vi "Write Data Container.vi"(8 "error in (no error)":errorcluster, 10 "Data Container":T1 {"WaveformData"."StopTime" format="%<%x %.3X>T"; "WaveformData"."StartTime" format="%<%x %.3X>T"}, 11 "Task_Abstr in":refnum<class "Task_Abstr.lvclass">) -> (0 "error out":errorcluster, 3 "Task_Abstr out":refnum<class "Task_Abstr.lvclass">)   [LabVIEW 2025, in "Task_Abstr.lvlib" / "Task_Abstr.lvclass"]
uses:
  Task_Abstr.lvclass
  DataContainer.ctl
  WaveformData.ctl
  Task_Abstr.lvclass/Task_Abstr.ctl
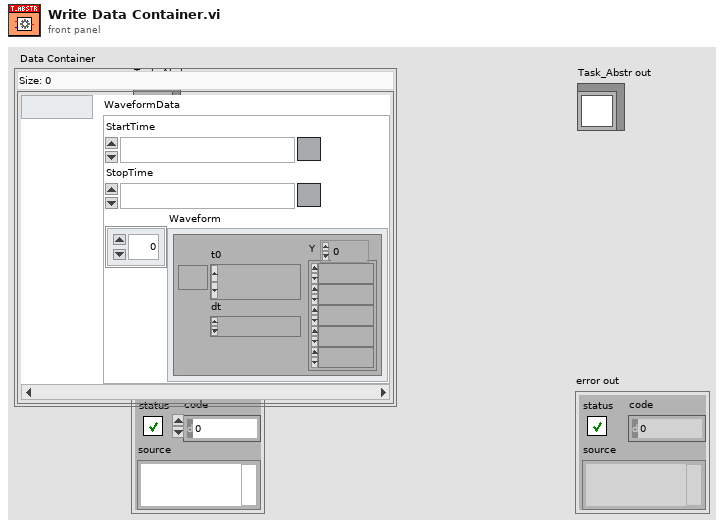
[diagram p1: front panel]
types:
  T1 = typedef "Task_Abstr.lvlib/Task_Abstr.lvclass/DataContainer.ctl" = map{string, T2}
  T2 = typedef "Task_Abstr.lvlib/Task_Abstr.lvclass/WaveformData.ctl" = cluster{"StartTime":timestamp, "StopTime":timestamp, "Waveform":waveform(dbl)[]}
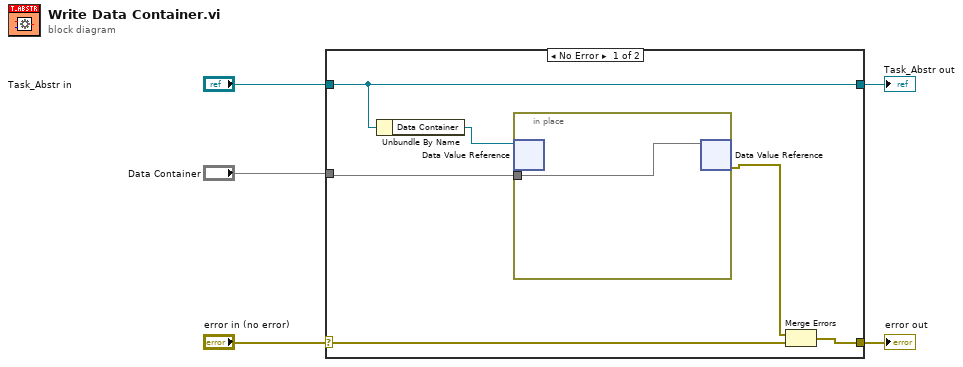
[diagram p0: block diagram]
diagram:
  n1 = case shown="No Error" "error in (no error)" {
    selector: "error in (no error)" -> [w7 w13]
    tunnel: [w8 w13] -> w4
    tunnel: [w11 w14] -> w2
    tunnel: "Task_Abstr in" -> [w11 w14]
    tunnel: "Data Container" -> [w9 _]
    frame No Error {
      n2 = Unbundle By Name(w11) -> ("Data Container"=w10:refnum<data-value>)
      n3 = in-place {
        in-place-border: w9 -> [w12]
        n4 = in-place-dvr #1(w10) -> ()  [unwired: 2 out]
        n5 = in-place-dvr #1(w12) -> (w6:errorcluster)  [unwired: 1 out]
      }
      n6 = Merge Errors(w6, w7) -> (w8:errorcluster)
    }
    frame Error {
    }
  }
  "error out" <- w4
  "Task_Abstr out" <- w2
